vi "Configure Bus Definition (Single Bit).vi"(7 "Enable Bit Display (T: Enable)":bool=TRUE, 8 "error in (no error)":errorcluster, 9 "Bit Position (0: Bit 0)":i32(ring) items=["Bit 0", "Bit 1", "Bit 2", "Bit 3", "Bit 4", "Bit 5", "Bit 6", "Bit 7", "Bit 8", "Bit 9", "Bit 10", "Bit 11", "Bit 12", "Bit 13", "Bit 14", "Bit 15"], 10 "Bus Name (1: Digital Bus 1)":i32(ring)=1 items=["Digital Bus 1"=1, "Digital Bus 2"=2], 11 "VISA resource name":refnum<visa-resource-name>) -> (0 "error out":errorcluster, 3 "VISA resource name out":refnum<visa-resource-name>)   [LabVIEW 2016, in "Agilent 2000 3000 X-Series.lvlib"]
doc: "Configures the digital bus definition in single bit mode. \n\n<B>Note(s):</B>\nThis function is only valid for the MSO models."
uses:
  Agilent 2000 3000 X-Series.lvlib
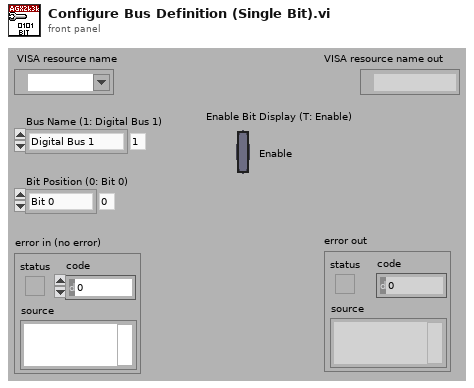
[diagram p1: front panel]
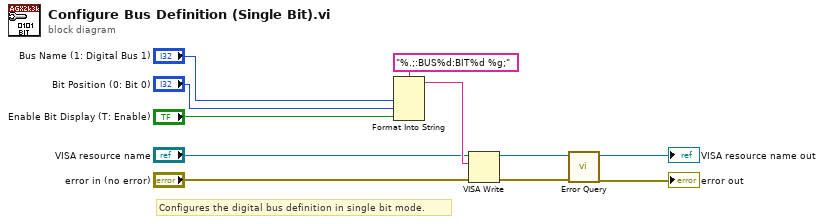
[diagram p0: block diagram]
diagram:
  # "Configures the digital bus definition in single bit mode."
  n1 = Format Into String(format string="%.;:BUS%d:BIT%d %g;", "Bus Name (1: Digital Bus 1)", "Bit Position (0: Bit 0)", "Enable Bit Display (T: Enable)") -> (resulting string=w9:string)  [unwired: 2 in, 1 out]
  n2 = VISA Write(VISA resource name="VISA resource name", write buffer=w9, error in (no error)="error in (no error)") -> (VISA resource name out=w6:refnum<visa-resource-name>, error out=w5:errorcluster)  [unwired: 1 out]
  n3 = call "Error Query.vi"("error in (no error)"=w5, "VISA resource name"=w6) -> ("error out"=→"error out":errorcluster, "VISA resource name out"=→"VISA resource name out":refnum<visa-resource-name>)  [unwired: 8 out]
